vi "Translator.TranslateThis.Init.vi"(8 "error in":errorcluster) -> (0 "error out":errorcluster)   [LabVIEW 2016]
uses:
  Config/Config.Global.vi
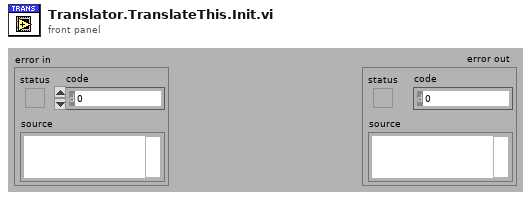
[diagram p1: front panel]
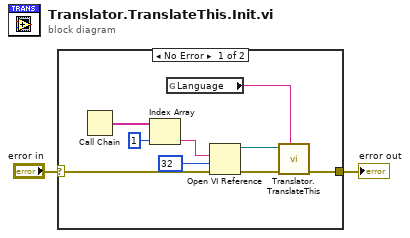
[diagram p0: block diagram]
diagram:
  n1 = case shown="No Error" "error in" {
    selector: "error in" -> [w4 w12]
    tunnel: [w11 w12] -> w2
    frame No Error {
      n2 = Call Chain() -> (call chain=w5:string[])
      n3 = Index Array(array=w5, index=1) -> (element=w9:string)
      n4 = global read "Config.Global.vi" "Language"() -> (w10:string)
      n5 = Open VI Reference(vi path=w9, options=32, error in (no error)=w4) -> (vi reference=w7:refnum<vi>, error out=w6:errorcluster)  [unwired: 1 in, 2 out]
      n6 = call "Translator.TranslateThis.vi"("Language (English)"=w10, "error in"=w6, "vi reference"=w7) -> ("error out"=w11:errorcluster)  [unwired: 8 in]
    }
    frame Error {
    }
  }
  "error out" <- w2
